vi "Write Speed.vi"(8 "error in (no error)":errorcluster, 10 "Speed":dbl[](array[numeric]), 11 "Motion Controller in":refnum<class "Motion Controller.lvclass">) -> (0 "error out":errorcluster, 3 "Motion Controller out":refnum<class "Motion Controller.lvclass">)   [LabVIEW 2022 SP3, in "Motion Controller.lvclass"]
uses:
  Motion Controller.lvclass
  Motion Controller.lvclass/Motion Controller.ctl
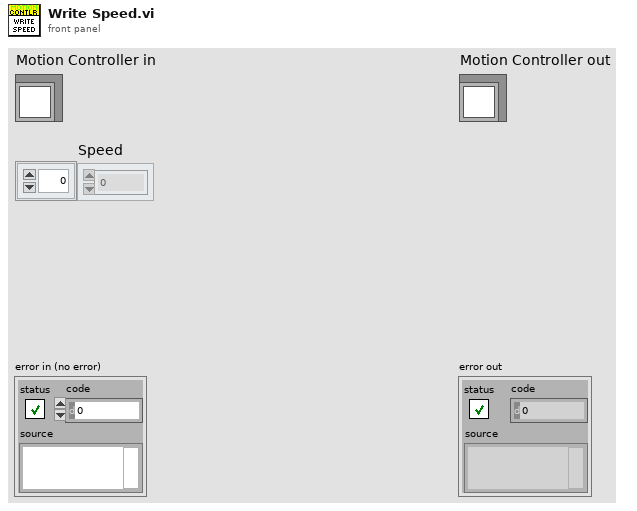
[diagram p1: front panel]
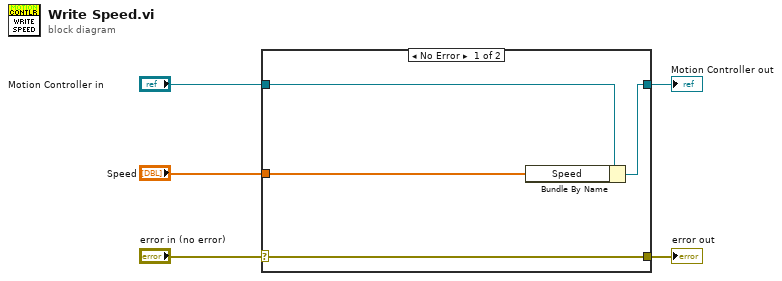
[diagram p0: block diagram]
diagram:
  n1 = case shown="No Error" "error in (no error)" {
    selector: "error in (no error)" -> [w9 w10]
    tunnel: [w9 w10] -> w4
    tunnel: [w7 w11] -> w2
    tunnel: "Motion Controller in" -> [w8 w11]
    tunnel: "Speed" -> [w6 _]
    frame No Error {
      n2 = Bundle By Name(cluster=w8, "Speed"=w6) -> (w7:refnum<class "Motion Controller.lvclass">)
    }
    frame Error {
    }
  }
  "error out" <- w4
  "Motion Controller out" <- w2
